vi "convertToTable.vi"(8 "error in (no error)":errorcluster, 11 "simonMessages in":refnum<class "simonMessages.lvclass">) -> (0 "error out":errorcluster, 2 "Message table":string[][](array[string]), 3 "simonMessages out":refnum<class "simonMessages.lvclass">)   [LabVIEW 2020, in "simonMessages.lvclass"]
uses:
  simonMessages.lvclass
  simonMessages.lvclass/simonMessages.ctl
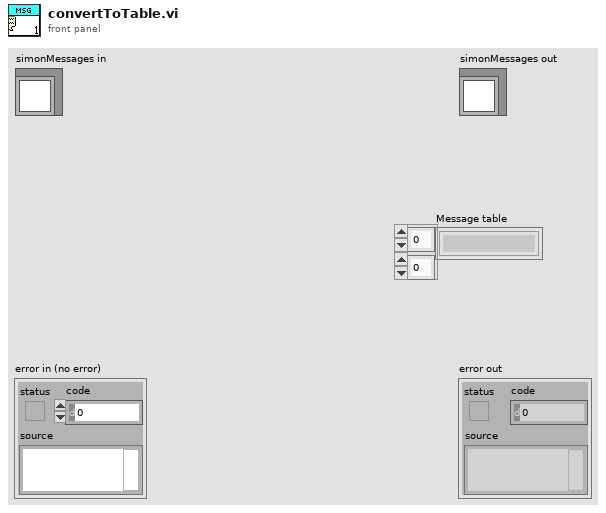
[diagram p1: front panel]
types:
  T1 = map{string, cluster{"Text":string, "Size":u8, "Justification":enum16{"Left", "Center", "Right"}, "Display Type":string}}
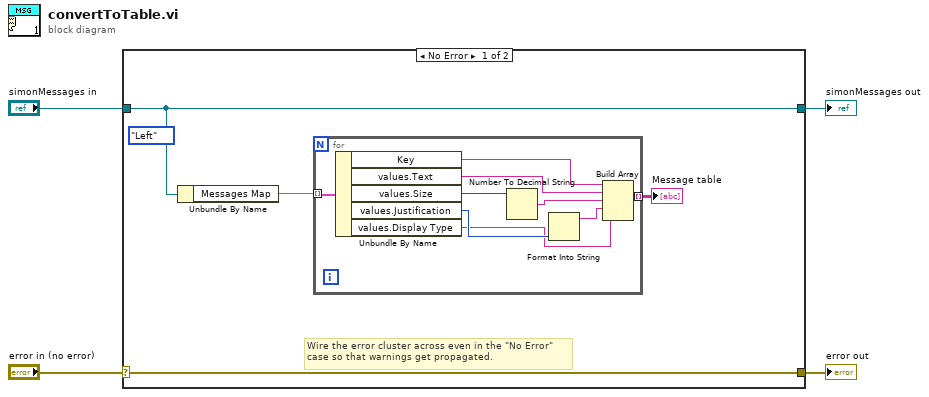
[diagram p0: block diagram]
diagram:
  n1 = case shown="No Error" "error in (no error)" {
    selector: "error in (no error)" -> [w8 w19]
    tunnel: [w8 w19] -> w3
    tunnel: [w7 w18] -> w1
    tunnel: "simonMessages in" -> [w7 w18]
    frame No Error {
      (unwired) enum16{"Left", "Center", "Right"}."Left" ("values.Justification")
      # "Wire the error cluster across even in the \"No Error\"\ncase so that warnings get propagated."
      n2 = Unbundle By Name(w7) -> ("Messages Map"=w6:T1)
      n3 = for {
        tunnel: w6 -> [w17] mode=indexing
        tunnel: [w12] -> w5 mode=indexing
        n4 = Unbundle By Name(w17) -> ("Key"=w14:string, "values.Text"=w13:string, "values.Size"=w16:u8, "values.Justification"=w15:enum16{"Left", "Center", "Right"}, "values.Display Type"=w9:string)
        n5 = Number To Decimal String(number=w16) -> (decimal integer string=w11:string)  [unwired: 1 in]
        n6 = Format Into String(w15) -> (resulting string=w10:string)  [unwired: 3 in, 1 out]
        n7 = Build Array(w14, w13, w11, w10, w9) -> (w12:string[])
      }
      "Message table" <- w5
    }
    frame Error {
    }
  }
  "error out" <- w3
  "simonMessages out" <- w1
